vi "Try Finalize Video.vi"(8 "error in (no error)":errorcluster, 11 "SB App in":refnum<class "SB App.lvclass">) -> (0 "error out":errorcluster, 3 "SB App out":refnum<class "SB App.lvclass">)   [LabVIEW 2020, in "SB App.lvlib" / "SB App.lvclass"]
uses:
  SB App.lvclass
  SB App.lvclass/SB App.ctl
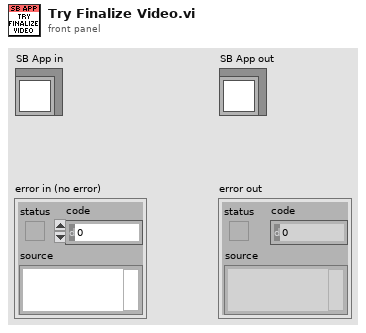
[diagram p1: front panel]
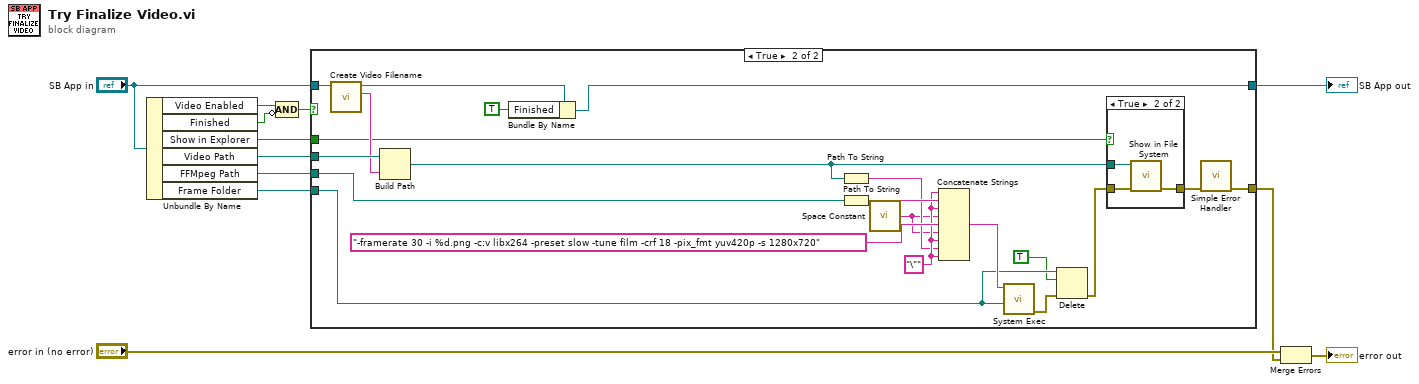
[diagram p0: block diagram]
diagram:
  n1 = Unbundle By Name("SB App in") -> ("Video Enabled"=w3:bool, "Finished"=w2:bool, "Show in Explorer"=w4:bool, "Video Path"=w11:path, "FFMpeg Path"=w10:path, "Frame Folder"=w7:path)
  n2 = Compound Arithmetic op=AND(w3, invert w2) -> (w1:bool)
  n3 = case shown="True" w1 {
    tunnel: w11 -> [_ w33]
    tunnel: w10 -> [_ w31]
    tunnel: "SB App in" -> [w13 w34]
    tunnel: [w13 w15] -> w8
    tunnel: w7 -> [_ w24]
    tunnel: [_ w16] -> w5
    tunnel: w4 -> [_ w18]
    frame False {
    }
    frame True {
      w28 = "\"" ("string")
      n4 = call "Create Video Filename.vi"("SB App in"=w34) -> ("Video Filename"=w32:string, "SB App out"=w20:refnum<class "SB App.lvclass">)  [unwired: 8 in, 1 out]
      n5 = Build Path(base path=w33, name or relative path=w32) -> (appended path=w22:path)
      n6 = Bundle By Name(cluster=w20, "Finished"=TRUE) -> (w15:refnum<class "SB App.lvclass">)
      n7 = Path To String(path=w22) -> (string=w27:string)
      n8 = Path To String(path=w31) -> (string=w30:string)
      n9 = call <vilib>:"Space Constant.vi"() -> ("String"=w19:string)
      n10 = Concatenate Strings(w28, w30, w28, w19, "-framerate 30 -i %d.png -c:v libx264 -preset slow -tune film -crf 18 -pix_fmt yuv420p -s 1280x720", w19, w28, w27, w28) -> (w26:string)
      n11 = call <vilib>:"System Exec.vi"("working directory"=w24, "command line"=w26) -> ("error out"=w25:errorcluster)  [unwired: 6 in, 3 out]
      n12 = Delete(path (use dialog)=w24, entire hierarchy (F)=TRUE, error in=w25) -> (error out=w21:errorcluster)  [unwired: 2 in, 2 out]
      n13 = case shown="True" w18 {
        tunnel: w22 -> [_ w38]
        tunnel: w21 -> [w35 w37]
        tunnel: [w35 w36] -> w17
        frame False {
        }
        frame True {
          n14 = call <vilib>:"Show in File System.vi"("error in (no error)"=w37, "file or directory path"=w38) -> ("error out"=w36:errorcluster)  [unwired: 9 in]
        }
      }
      n15 = call <vilib>:"Simple Error Handler.vi"("error in (no error)"=w17) -> ("error out"=w16:errorcluster)  [unwired: 4 in, 4 out]
    }
  }
  "SB App out" <- w8
  n16 = Merge Errors("error in (no error)", w5) -> (→"error out":errorcluster)
